vi "Update Comb and BW Control Visibility.vi"(5 "Filter response":u32(ring) items=["Comb"=0, "Butterworth"=2], 7 "Butterworth filter order":refnum<vi>, 8 "Butterworth cutoff frequency":refnum<vi>, 9 "comb frequency":refnum<vi>) -> ()   [LabVIEW 2017, in "Modules.lvlib" / "9253.lvclass"]
uses:
  9253.lvclass
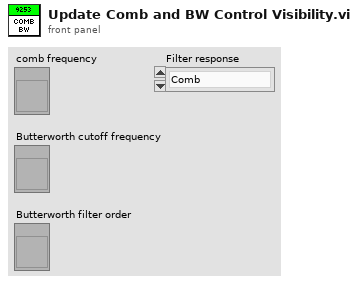
[diagram p1: front panel]
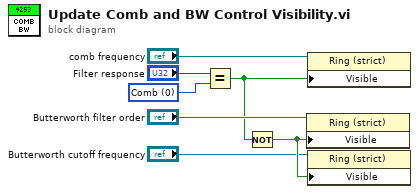
[diagram p0: block diagram]
diagram:
  w2 = u32 0 items=["Comb"=0, "Butterworth"=2] ("Filter response")
  n1 = Equal?(x="Filter response", y=w2) -> (x = y?=w3:bool)
  n2 = Not(x=w3) -> (.not. x?=w6:bool)
  n3 = property class="Ring (strict)"(reference="Butterworth filter order", "Visible"=w6) -> ()  [unwired: 1 in, 2 out]
  n4 = property class="Ring (strict)"(reference="comb frequency", "Visible"=w3) -> ()  [unwired: 1 in, 2 out]
  n5 = property class="Ring (strict)"(reference="Butterworth cutoff frequency", "Visible"=w6) -> ()  [unwired: 1 in, 2 out]
